vi "Set Brightness.vi"(8 "error in (no error)":errorcluster, 9 "Brightness":i32(slide) scale=3.0..100.0, 10 "Light Selection":T1, 11 "LightsPanel in":refnum<class "LightsPanel.lvclass">) -> (0 "error out":errorcluster, 3 "LightsPanel out":refnum<class "LightsPanel.lvclass">)   [LabVIEW 2022 SP3, in "TouchControl.lvlib" / "LightsPanel.lvclass"]
uses:
  LightsPanel.lvclass
  Light Selection.ctl
  LightsPanel.lvclass/LightsPanel.ctl
  Update Type.ctl
  TouchControl.lvlib
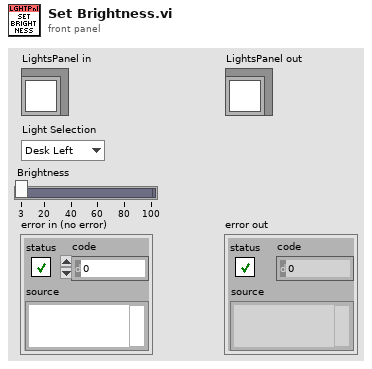
[diagram p1: front panel]
types:
  T1 = typedef "TouchControl.lvlib/Light Selection.ctl" = enum16{"Desk Left", "Desk Right", "Printer"}
  T2 = typedef "TouchControl.lvlib/LightsPanel.lvclass/Update Type.ctl" = enum16{"Light On", "Temp", "Brightness"}
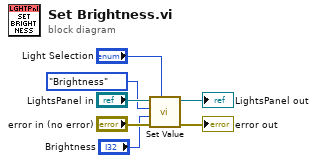
[diagram p0: block diagram]
diagram:
  n1 = call "Set Value.vi"("Light Selection"="Light Selection", "error in (no error)"="error in (no error)", "Value"="Brightness", "Update Type"=Update_Type."Brightness", "LightsPanel in"="LightsPanel in") -> ("error out"=→"error out":errorcluster, "LightsPanel out"=→"LightsPanel out":refnum<class "LightsPanel.lvclass">)  [unwired: 5 in]
